vi "launch_dynamic_vi.vi"(7 "queue":T2, 8 "error in (no error)":errorcluster, 10 "cycle":i32, 11 "profile":T1[](array[typedef])) -> (0 "error out":errorcluster)   [LabVIEW 2019]
uses:
  core_dataRefCluster.ctl
  core_dataRef.ctl
  core_dataCluster.ctl
  core_setup.ctl
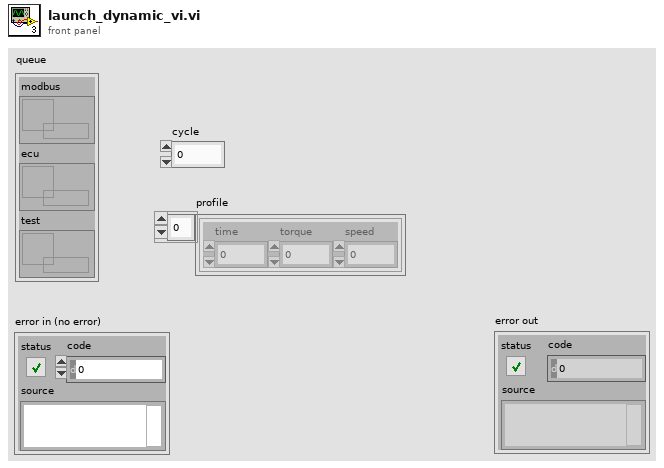
[diagram p1: front panel]
types:
  T1 = typedef "core_setup.ctl" = cluster{"time":i32, "torque":dbl, "speed":i32}
  T2 = typedef "core_dataRefCluster.ctl" = cluster{"modbus":T3, "ecu":T3, "test":T3}
  T3 = typedef "core_dataRef.ctl" = refnum<queue>
  T4 = enum32{"Bad", "Idle", "Run top level", "Running"}
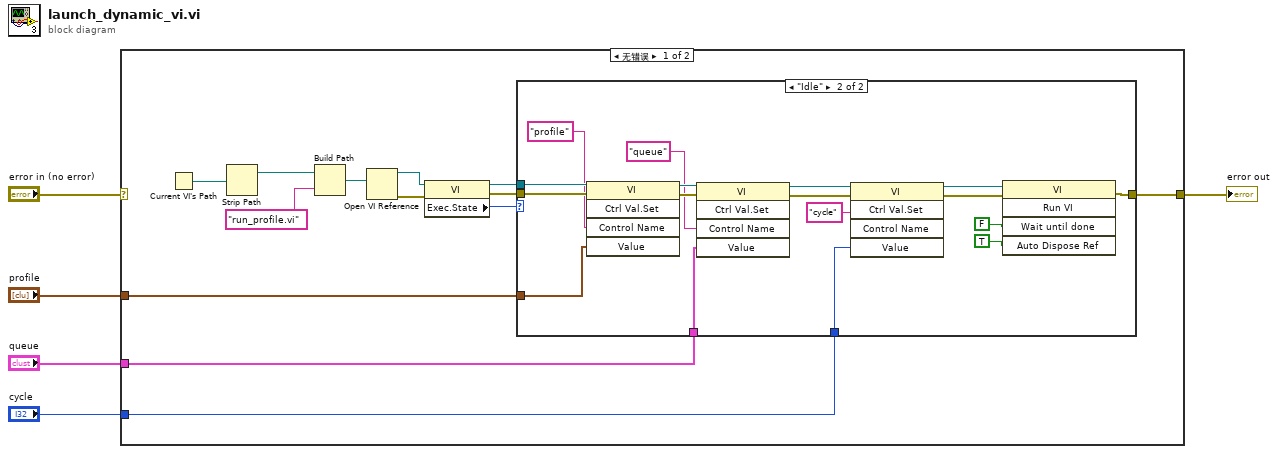
[diagram p0: block diagram]
diagram:
  n1 = case shown="无错误" "error in (no error)" {
    selector: "error in (no error)" -> [_ w37]
    tunnel: "profile" -> [w9 _]
    tunnel: [w8 w37] -> w4
    tunnel: "queue" -> [w7 _]
    tunnel: "cycle" -> [w6 _]
    frame No Error {
      n2 = Current VI's Path() -> (path=w18:path)
      n3 = Strip Path(path=w18) -> (stripped path=w17:path)  [unwired: 1 out]
      n4 = Build Path(base path=w17, name or relative path="run_profile.vi") -> (appended path=w15:path)
      n5 = Open VI Reference(vi path=w15) -> (vi reference=w14:refnum<vi>, error out=w13:errorcluster)  [unwired: 5 in]
      n6 = property class="VI"(reference=w14, error in=w13) -> (reference out=w11:refnum<vi>, error out=w10:errorcluster, "Exec.State"=w12:T4)
      n7 = case shown="\"Idle\"" w12 {
        tunnel: w11 -> [_ w36]
        tunnel: w10 -> [w19 w34]
        tunnel: w9 -> [_ w31]
        tunnel: [w19 w30] -> w8
        tunnel: w7 -> [_ w27]
        tunnel: w6 -> [_ w20]
        frame "Bad", Default {
        }
        frame "Idle" {
          n8 = invoke class="VI" method="Ctrl Val.Set"(reference=w36, error in=w34, "Control Name"="profile", "Value"=w31) -> (reference out=w35:refnum<vi>, error out=w33:errorcluster)  [unwired: 1 in, 3 out]
          n9 = invoke class="VI" method="Ctrl Val.Set"(reference=w35, error in=w33, "Control Name"="queue", "Value"=w27) -> (reference out=w32:refnum<vi>, error out=w23:errorcluster)  [unwired: 1 in, 3 out]
          n10 = invoke class="VI" method="Ctrl Val.Set"(reference=w32, error in=w23, "Control Name"="cycle", "Value"=w20) -> (reference out=w24:refnum<vi>, error out=w22:errorcluster)  [unwired: 1 in, 3 out]
          n11 = invoke class="VI" method="Run VI"(reference=w24, error in=w22, "Wait until done"=FALSE ("Wait Until Done"), "Auto Dispose Ref"=TRUE ("Auto Dispose Reference")) -> (error out=w30:errorcluster)  [unwired: 1 in, 4 out]
        }
      }
    }
    frame Error {
    }
  }
  "error out" <- w4
